vi "StringQueueRef.vi"(11 "String Queue Refnum":refnum<queue>) -> (2 "Display String":string, 3 "Stop?":bool)   [LabVIEW 2020]
doc: "Displays the queue name, the elements of the queue, the number of elements in the queue, the number of pending insert items, the number of pending remove items, and the hex value of the reference. You can use this probe to set a breakpoint if the value is an invalid refnum."
uses:
  <vilib>/Utility/error.llb/DialogTypeEnum.ctl
panel:
  in  "Unnamed":string="Unnamed"
  in  "error source":string="Sring Queue Refnum Probe"
  in  "number pending remove":string="Number pending remove"
  in  "number of elements":string="Number of elements"
  in  "queue name":string="Queue name"
  in  "number pending insert":string="Number pending insert"
  in  "Pause if Not a Refnum":bool
  out "Elements":string[](array[string])
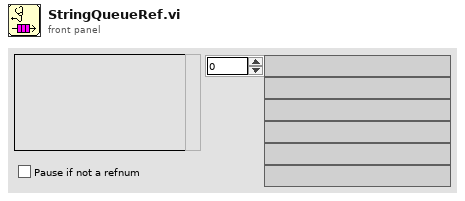
[diagram p1: front panel]
types:
  T1 = typedef "DialogTypeEnum.ctl" = enum16{"no dialog", "OK message", "continue or stop message", "auto error handling dialog", "OK message + warnings", "continue/stop + warnings"}
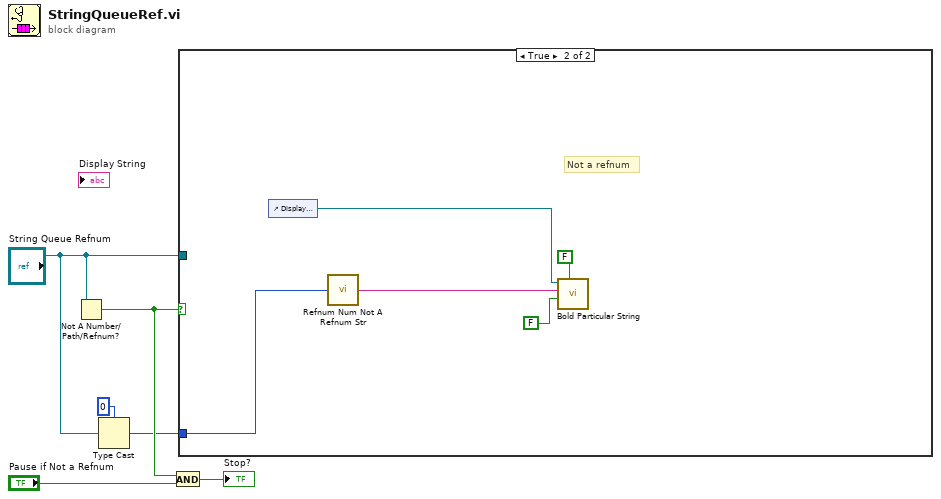
[diagram p0: block diagram]
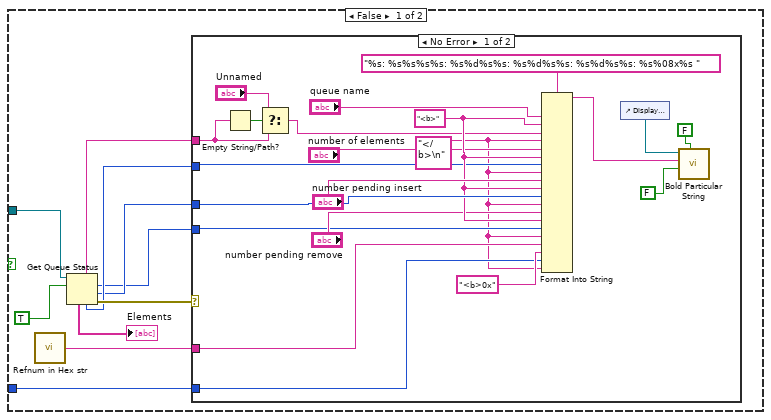
[diagram p2: hidden frame]
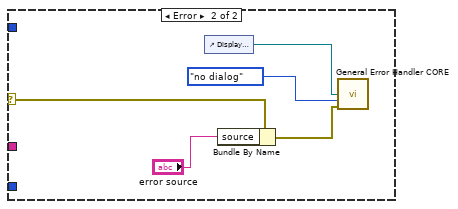
[diagram p3: hidden frame]
diagram:
  n1 = Not A Number/Path/Refnum?(number/path/refnum="String Queue Refnum") -> (NaN/Path/Refnum?=w4:bool)
  n2 = Type Cast(type=u32 0, x="String Queue Refnum") -> (*(type *) &x=w2:u32)
  n3 = And(x=w4, y="Pause if Not a Refnum") -> (x .and. y?=→"Stop?":bool)
  n4 = case shown="True" w4 {
    tunnel: "String Queue Refnum" -> [w14 _]
    tunnel: w2 -> [w8 w43]
    frame False {
      n5 = call <vilib>:"Refnum in Hex str.vi"() -> ("refnum in hex"=w9:string)
      n6 = Get Queue Status(queue=w14, return elements? (F)=TRUE) -> (queue name=w15:string, # pending remove=w11:i32, # pending insert=w12:i32, error out=w16:errorcluster, # elements in queue=w13:i32, elements=→"Elements":string[])  [unwired: 1 in, 2 out]
      n7 = case shown="No Error" w16 {
        selector: w16 -> [_ w41]
        tunnel: w15 -> [w19 _]
        tunnel: w8 -> [w29 _]
        tunnel: w9 -> [w31 _]
        tunnel: w13 -> [w23 _]
        tunnel: w12 -> [w35 _]
        tunnel: w11 -> [w32 _]
        frame No Error {
          w22 = "</b>\n"
          w34 = "<b>"
          n8 = Empty String/Path?(string/path=w19) -> (empty?=w20:bool)
          n9 = Select(t="Unnamed", s=w20, f=w19) -> (s? t:f=w17:string)
          n10 = Format Into String(format string="%s: %s%s%s%s: %s%d%s%s: %s%d%s%s: %s%d%s%s: %s%08x%s ", "queue name", w34, w17, w22, "number of elements", w34, w23, w22, "number pending insert", w34, w35, w22, "number pending remove", w34, w32, w22, w31, "<b>0x", w29, w22) -> (resulting string=w27:string)  [unwired: 2 in, 1 out]
          n11 = control-ref of="Display String"() -> (w28:refnum<vi>)
          n12 = call <vilib>:"Bold Particular String.vi"("Always Refresh? (TRUE)"=FALSE ("Always Refresh? (FALSE)"), "resize string? (TRUE)"=FALSE, "text to display"=w27, "string refnum"=w28) -> ()  [unwired: 6 in, 2 out]
        }
        frame Error {
          n13 = control-ref of="Display String"() -> (w39:refnum<vi>)
          n14 = Bundle By Name(cluster=w41, "source"="error source") -> (w40:errorcluster)
          n15 = call <vilib>:"General Error Handler CORE.vi"("String to Format (not a refnum)"=w39, "type of dialog (OK msg:1)"=DialogTypeEnum."no dialog", "error in (no error)"=w40) -> ()  [unwired: 7 in, 6 out]
        }
      }
    }
    frame True {
      # "Not a refnum"
      n16 = control-ref of="Display String"() -> (w47:refnum<vi>)
      n17 = call <vilib>:"Refnum Num Not A Refnum Str.vi"("Numeric"=w43) -> ("text to display"=w44:string)
      n18 = call <vilib>:"Bold Particular String.vi"("Always Refresh? (TRUE)"=FALSE ("Always Refresh? (FALSE)"), "resize string? (TRUE)"=FALSE, "text to display"=w44, "string refnum"=w47) -> ()  [unwired: 6 in, 2 out]
    }
  }
